vi "Configure Run Information.vi"(8 "error in":errorcluster, 11 "App Data In":T1) -> (0 "error out":errorcluster, 3 "App Data Out":T1)   [LabVIEW 2021]
uses:
  Controls/App Data Cluster.ctl
panel:
  in  "Ok":bool
  in  "Unit":string
  in  "Device location":string
  in  "Sensor type":string
  in  "Device name":string
  in  "Device ID":dbl
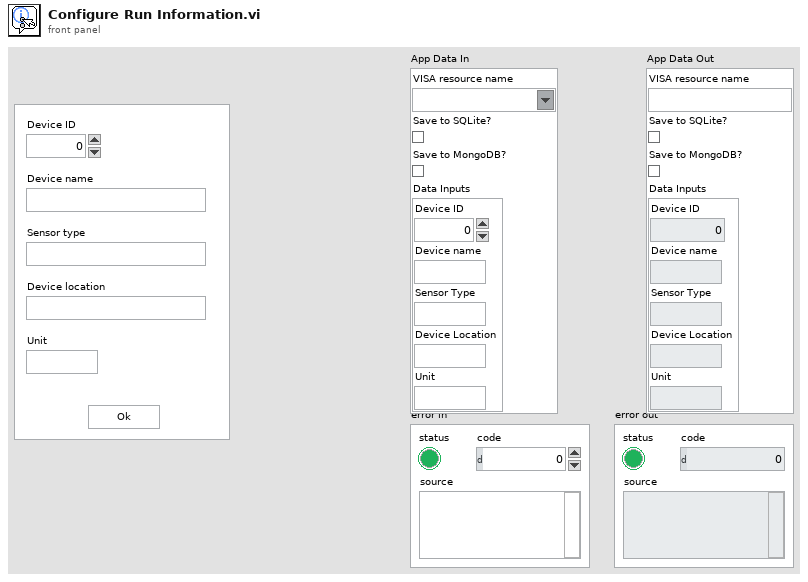
[diagram p1: front panel]
types:
  T1 = typedef "App Data Cluster.ctl" = cluster{"VISA resource name":refnum<visa-resource-name>, "Save to SQLite?":bool, "Save to MongoDB?":bool, "Data Inputs":cluster{"Device ID":dbl, "Device name":string, "Sensor Type":string, "Device Location":string, "Unit":string}}
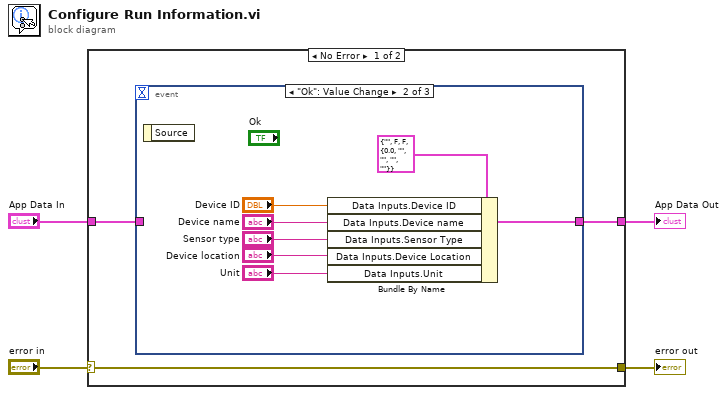
[diagram p0: block diagram]
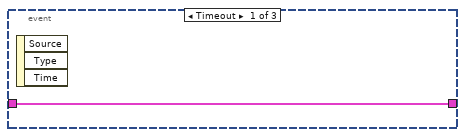
[diagram p2: hidden frame]
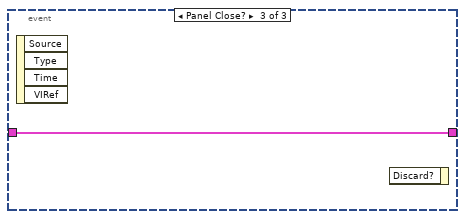
[diagram p3: hidden frame]
diagram:
  n1 = case shown="No Error" "error in" {
    selector: "error in" -> [w7 w18]
    tunnel: [w7 w18] -> w3
    tunnel: [w6 w17] -> w2
    tunnel: "App Data In" -> [w5 w17]
    frame No Error {
      n2 = event shown="[1] \"Ok\": Value Change" {
        selector: _ -> [_ _ _]
        dyn-events: _ -> [_ _ _]
        timeout: _ -> [_ _ _]
        tunnel: [w8 w9 w16] -> w6
        tunnel: w5 -> [w8 _ w16]
        event Timeout {
          n3 = event-data() -> ()  [unwired: 1 in, 3 out]
        }
        event "Ok": Value Change {
          n4 = event-data() -> ()  [unwired: 1 in, 1 out]
          n5 = Bundle By Name(cluster=T1 {"VISA resource name"="", "Save to SQLite?"=FALSE, "Save to MongoDB?"=FALSE, "Data Inputs"={"Device ID"=0.0, "Device name"="", "Sensor Type"="", "Device Location"="", "Unit"=""}} ("App Data"), "Data Inputs.Device ID"="Device ID", "Data Inputs.Device name"="Device name", "Data Inputs.Sensor Type"="Sensor type", "Data Inputs.Device Location"="Device location", "Data Inputs.Unit"="Unit") -> (w9:T1)
        }
        event Panel Close? {
          n6 = event-data() -> ()  [unwired: 1 in, 4 out]
          n7 = event-data() -> ()  [unwired: 2 in, 1 out]
        }
      }
    }
    frame Error {
    }
  }
  "error out" <- w3
  "App Data Out" <- w2
